vi "XiXi-1(XOR Boolean[]).vi"(10 "X[-1]":bool[](array[boolean]), 11 "Xi":bool[][](array[boolean])) -> (3 "Yi":bool[][](array[boolean]))   [LabVIEW 2012]
doc: "Calculate sums of consecutive array elements. 0th element of output is equal to x(0)+ x(-1), where x(-1) is an optional scalar input that defaults to zero."
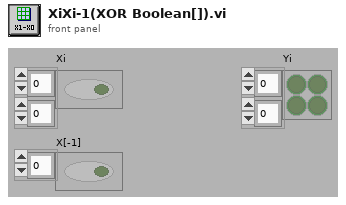
[diagram p1: front panel]
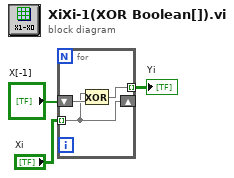
[diagram p0: block diagram]
diagram:
  n1 = for {
    shift-right: [w5] -> _
    shift-left: "X[-1]" -> [w6]
    tunnel: "Xi" -> [w5] mode=indexing
    tunnel: [w4] -> w1 mode=indexing
    n2 = Exclusive Or(1:w6, 2:w5) -> (0:w4:bool[])
  }
  "Yi" <- w1
